vi "MinDistanceToObstaclewAng.vi"(8 "error in (no error)":errorcluster, 10 "Boat":T1 {"North" format="%#_10f"; "East" format="%#_8f"}, 11 "Obstacle.lvclass":refnum<class "Obstacle.lvclass">) -> (0 "Closest point to boat":T1 {"North" format="%#_10f"; "East" format="%#_8f"}, 1 "Min angle (deg)":dbl, 2 "Min angle (rad)":dbl, 3 "Min distance":dbl)   [LabVIEW 2013, in "Obstacle.lvclass"]
uses:
  Obstacle.lvclass
  Data/TypeDefs/UTM Location.ctl
  Obstacle.lvclass/Obstacle.ctl
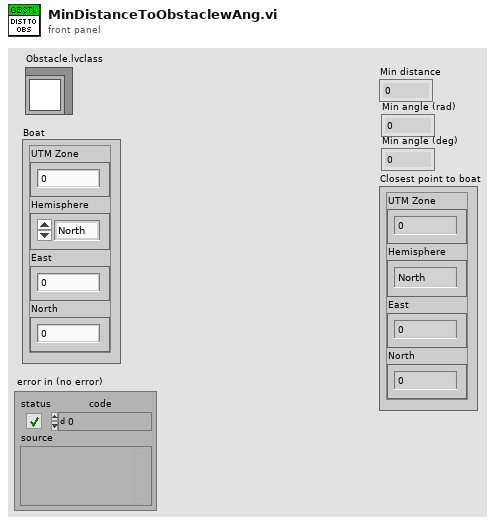
[diagram p1: front panel]
types:
  T1 = typedef "UTM Location.ctl" = cluster{"UTM Zone":dbl, "Hemisphere":enum16{"North", "South"}, "East":dbl, "North":dbl}
  T2 = cluster{"UTM Obstacle Point 2":T1, "UTM Obstacle Point 1":T1}[]
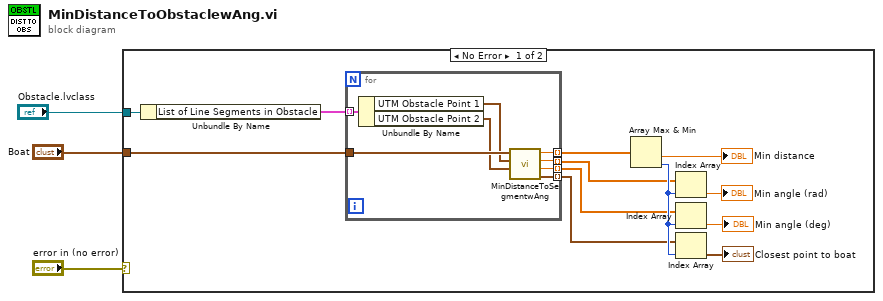
[diagram p0: block diagram]
diagram:
  n1 = case shown="No Error" "error in (no error)" {
    tunnel: "Obstacle.lvclass" -> [w15 _]
    tunnel: "Boat" -> [w13 _]
    frame No Error {
      n2 = Unbundle By Name(w15) -> ("List of Line Segments in Obstacle"=w14:T2)
      n3 = for {
        tunnel: w14 -> [w23] mode=indexing
        tunnel: w13 -> [w22]
        tunnel: [w19] -> w12 mode=indexing
        tunnel: [w18] -> w9 mode=indexing
        tunnel: [w17] -> w8 mode=indexing
        tunnel: [w16] -> w7 mode=indexing
        n4 = Unbundle By Name(w23) -> ("UTM Obstacle Point 1"=w21:T1, "UTM Obstacle Point 2"=w20:T1)
        n5 = call "MinDistanceToSegmentwAng.vi"("Segment Point 2"=w20, "Segment Point 1"=w21, "Boat Point"=w22) -> ("Closest point to boat"=w16:T1, "Angle to Obstacle, Trig Abs (deg)"=w17:dbl, "Angle to Obstacle, Trig Abs (rad)"=w18:dbl, "Distance between boat and segment"=w19:dbl)  [unwired: 5 in]
      }
      n6 = Array Max & Min(array=w12) -> (min value=→"Min distance":dbl, min index (indices)=w10:i32)  [unwired: 2 out]
      n7 = Index Array(array=w9, index=w10) -> (element=→"Min angle (rad)":dbl)
      n8 = Index Array(array=w8, index=w10) -> (element=→"Min angle (deg)":dbl)
      n9 = Index Array(array=w7, index=w10) -> (element=→"Closest point to boat":T1)
    }
    frame Error {
    }
  }
